vi "Greatest Common Divisor of p&q (CDB).vi"(6 "tolerance type":u16(ring) items=["Absolute", "Relative"], 7 "tolerance":dbl, 8 "order of q":i32, 9 "q":cdb[](array[numeric]) format="%.2f", 10 "order of p":i32, 11 "p":cdb[](array[numeric]) format="%.2f") -> (0 "rest":cdb[](array[numeric]) format="%.2f", 2 "coprime?":bool, 3 "greatest common factor":cdb[](array[numeric]) format="%.2f")   [LabVIEW 2017, in "NI_AALPro.lvlib"]
doc: "Determine the Greatest Common Factor between two polynomials."
uses:
  <vilib>/Analysis/NI_AALPro.lvlib
  <vilib>/Analysis/polynomials.llb/Remove Zero Threshold Type.ctl
  <vilib>/Analysis/5stat.llb/RMS (DBL).vi
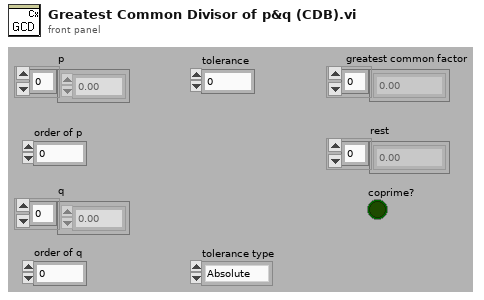
[diagram p1: front panel]
types:
  T1 = typedef "NI_AALPro.lvlib/Remove Zero Threshold Type.ctl" = u16
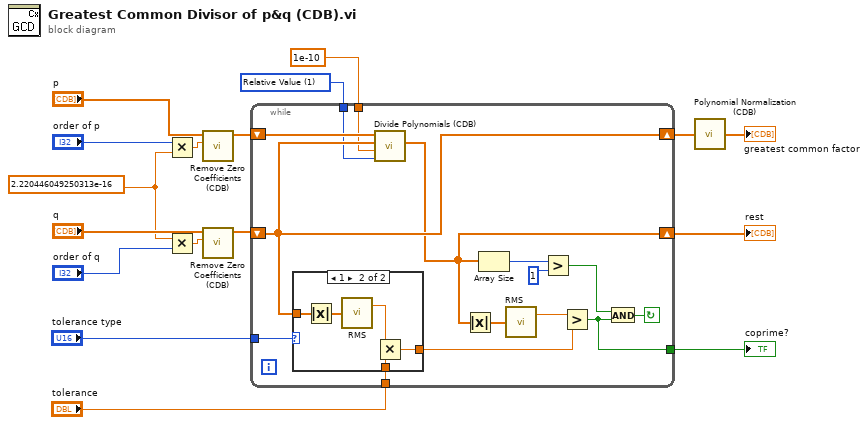
[diagram p0: block diagram]
diagram:
  w2 = T1 1 items=["Absolute Value", "Relative Value"] ("threshold type")
  w10 = 2.220446049250313e-16 ("eps for remove zeros")
  n1 = Multiply(x="order of p", y=w10) -> (x*y=w6:dbl)
  n2 = Multiply(x=w10, y="order of q") -> (x*y=w5:dbl)
  n3 = call <vilib>:"Remove Zero Coefficients (CDB).vi"("threshold"=w6, "P(x) In"="p") -> ("P(x) Out"=w16:cdb[])  [unwired: 7 in, 2 out]
  n4 = call <vilib>:"Remove Zero Coefficients (CDB).vi"("threshold"=w5, "P(x) In"="q") -> ("P(x) Out"=w15:cdb[])  [unwired: 7 in, 2 out]
  n5 = while {
    shift-left: w15 -> [w23]
    shift-right: [w20] -> w17
    shift-left: w16 -> [w32]
    shift-right: [w23] -> w9
    tunnel: "tolerance" -> [w24]
    tunnel: "tolerance type" -> [w25]
    tunnel: [w21] -> w3
    tunnel: w2 -> [w19]
    tunnel: 1e-10 ("threshold") -> [w18]
    stop <- w29 continue-if-true
    n6 = case shown="1" w25 {
      tunnel: w24 -> [w33 w34]
      tunnel: w23 -> [_ w38]
      tunnel: [w33 w36] -> w22
      frame 0, Default {
      }
      frame 1 {
        n7 = Absolute Value(x=w38) -> (abs(x)=w37:dbl[])
        n8 = call-poly <vilib>:"RMS.vi"("X"=w37) -> ("rms value"=w35:dbl)  [unwired: 1 out]
        n9 = Multiply(x=w35, y=w34) -> (x*y=w36:dbl)
      }
    }
    n10 = call <vilib>:"Divide Polynomials (CDB).vi"("threshold type"=w19, "threshold"=w18, "Q(x)"=w23, "P(x)"=w32) -> ("Remainder"=w20:cdb[])  [unwired: 5 in, 2 out]
    n11 = Absolute Value(x=w20) -> (abs(x)=w28:dbl[])
    n12 = Array Size(array=w20) -> (size(s)=w30:i32)
    n13 = call-poly <vilib>:"RMS.vi"("X"=w28) -> ("rms value"=w27:dbl)  [unwired: 1 out]
    n14 = Greater?(x=w30, y=1) -> (0:w26:bool)
    n15 = Greater?(x=w27, y=w22) -> (0:w21:bool)
    n16 = And(x=w26, y=w21) -> (x .and. y?=w29:bool)
  }
  "rest" <- w17
  "coprime?" <- w3
  n17 = call <vilib>:"Polynomial Normalization (CDB).vi"("polynomial"=w9) -> ("normalized polynomial"=→"greatest common factor":cdb[])
